vi "ReadData.vi"(2 "Error In":errorcluster, 3 "YINCrement":dbl=0.5, 4 "YOrigin":dbl, 5 "VISA resource name":refnum<visa-resource-name>) -> (0 "error out":errorcluster, 1 "Data":dbl[](array[numeric]))   [LabVIEW 2022 SP3]
panel:
  out "1st Character":string
  out "Waveform Graph":dbl[](graph)
  out "Data buffer":string
  out "Data Length":string
  out "Header Length":string
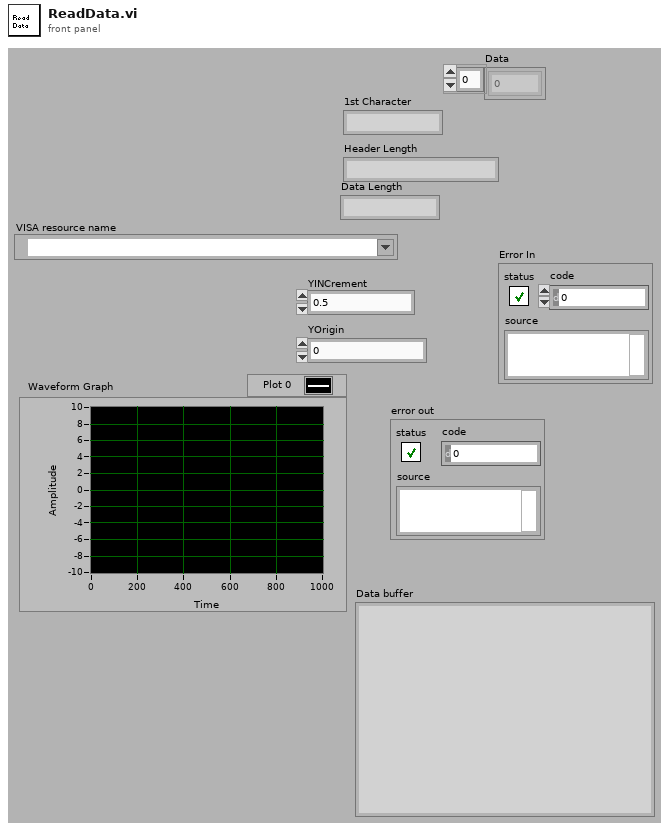
[diagram p1: front panel]
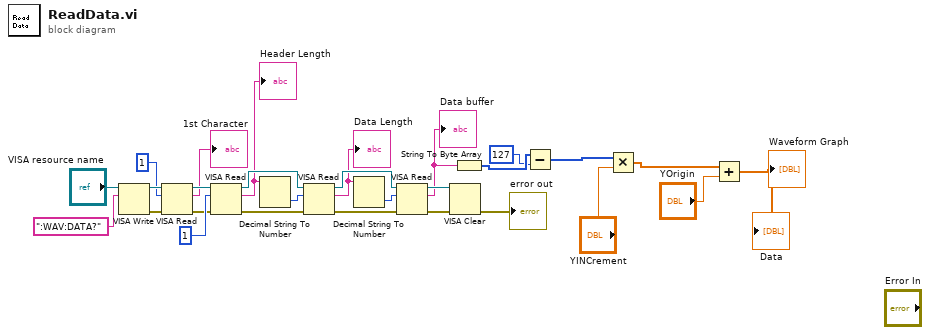
[diagram p0: block diagram]
diagram:
  n1 = VISA Write(VISA resource name="VISA resource name", write buffer=":WAV:DATA?") -> (VISA resource name out=w20:refnum<visa-resource-name>, error out=w19:errorcluster)  [unwired: 1 in, 1 out]
  n2 = VISA Read(VISA resource name=w20, byte count=u32 1, error in (no error)=w19) -> (VISA resource name out=w17:refnum<visa-resource-name>, read buffer=→"1st Character":string, error out=w16:errorcluster)  [unwired: 1 out]
  n3 = VISA Read(VISA resource name=w17, byte count=u32 1, error in (no error)=w16) -> (VISA resource name out=w24:refnum<visa-resource-name>, read buffer=w15:string, error out=w23:errorcluster)  [unwired: 1 out]
  "Header Length" <- w15
  n4 = Decimal String To Number(string=w15) -> (number=w14:i32)  [unwired: 2 in, 1 out]
  n5 = VISA Read(VISA resource name=w24, byte count=w14, error in (no error)=w23) -> (VISA resource name out=w22:refnum<visa-resource-name>, read buffer=w13:string, error out=w21:errorcluster)  [unwired: 1 out]
  "Data Length" <- w13
  n6 = Decimal String To Number(string=w13) -> (number=w12:i32)  [unwired: 2 in, 1 out]
  n7 = VISA Read(VISA resource name=w22, byte count=w12, error in (no error)=w21) -> (VISA resource name out=w11:refnum<visa-resource-name>, read buffer=w9:string, error out=w10:errorcluster)  [unwired: 1 out]
  "Data buffer" <- w9
  n8 = VISA Clear(VISA resource name=w11, error in (no error)=w10) -> (error out=→"error out":errorcluster)  [unwired: 1 out]
  n9 = String To Byte Array(string=w9) -> (unsigned byte array=w2:u8[])
  n10 = Subtract(x=w2, y=127 ("x")) -> (x-y=w6:i32[])
  n11 = Multiply(x=w6, y="YINCrement") -> (x*y=w4:dbl[])
  n12 = Add(x=w4, y="YOrigin") -> (x+y=→"Waveform Graph" →"Data":dbl[])
